vi "box viosion.vi"(8 "Error In":errorcluster) -> (0 "error out":errorcluster, 2 "Array out":string[][](array[string]))   [LabVIEW 2019]
panel:
  out "Array":cluster{i32, i32}[][](array[cluster])
  out "Image":T1(plugin-control)
  out "Image Out":T1(plugin-control)
  # "black\ngreen\nblue\nred"
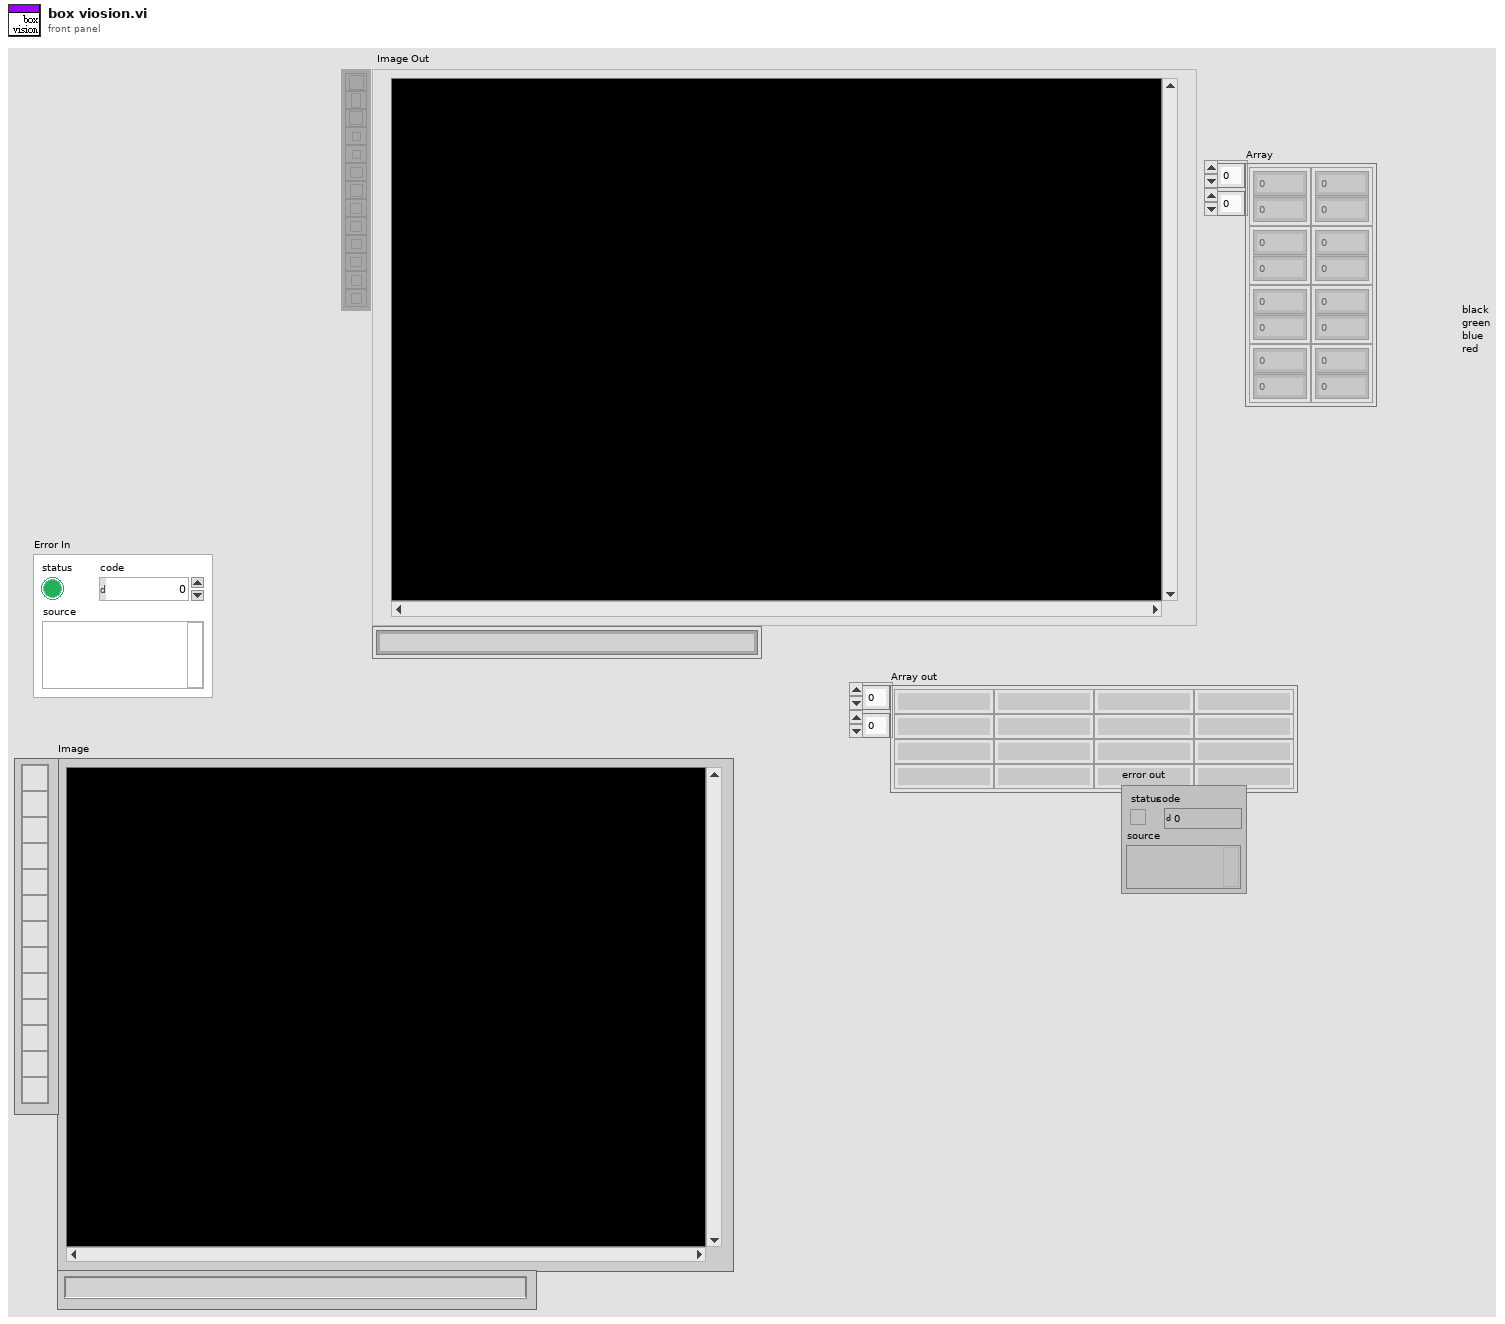
[diagram p1: front panel]
types:
  T1 = typedef "IMAQ Image.ctl" = refnum<image>
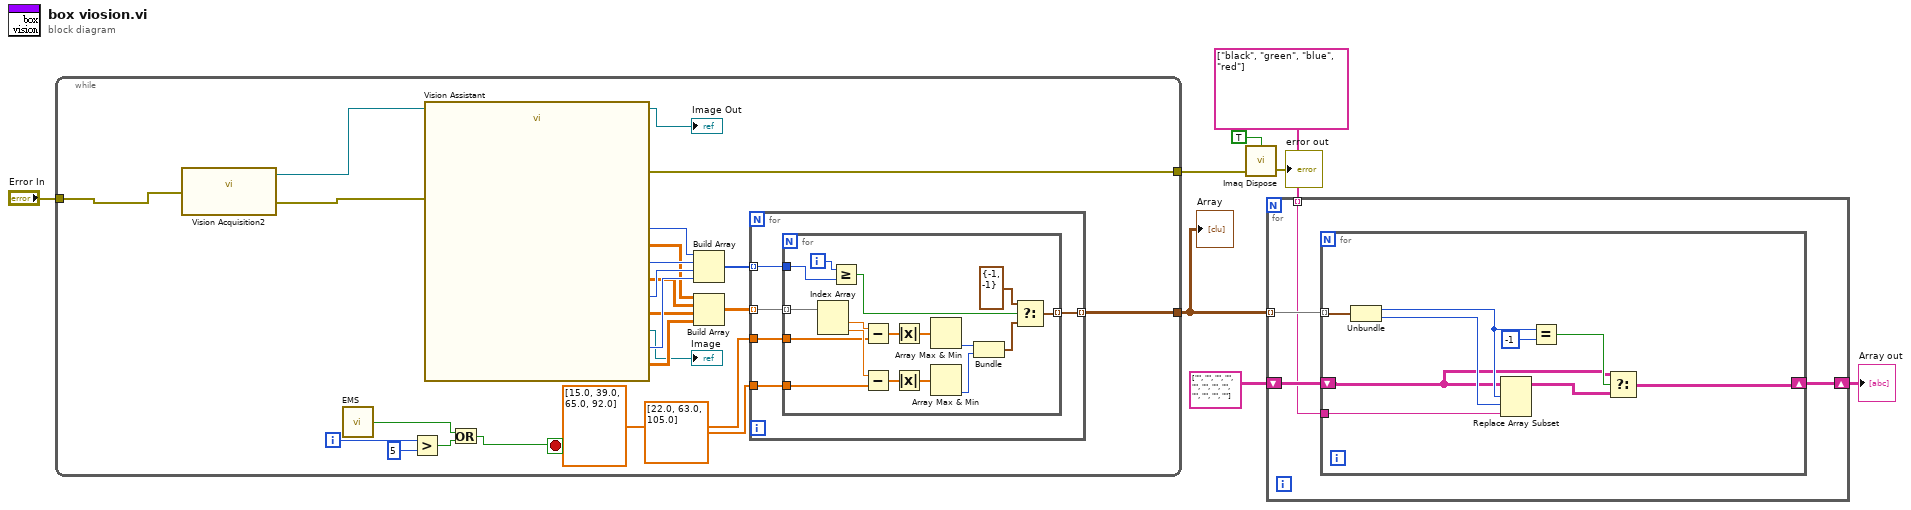
[diagram p0: block diagram]
diagram:
  n1 = while {
    tunnel: [w24] -> w1
    tunnel: "Error In" -> [w15]
    tunnel: [w18] -> w7
    i -> [w13]
    stop <- w9 stop-if-true
    n2 = call "Vision Acquisition2"("error in"=w15) -> ("Image Out"=w16:T1, "error out"=w14:errorcluster)  [unwired: 25 in]
    n3 = call "EMS.vi"() -> ("A/DIO4 (Pin 19)"=w10:bool)
    n4 = Greater?(x=w13, y=5) -> (0:w11:bool)
    n5 = call "Vision Assistant"("Image In"=w16, "error in"=w14) -> ("Image Buffer (Image Buffer 5)"=→"Image":T1, "Particle Measurements (Pixels) (Red)"=w26:dbl[][], "Number of Particles (Red)"=w31:i32, "Image Out"=→"Image Out":T1, "Number of Particles (Black)"=w32:i32, "Particle Measurements (Pixels) (Black)"=w28:dbl[][], "Number of Particles (Green)"=w29:i32, "Particle Measurements (Pixels) (Green)"=w27:dbl[][], "Number of Particles (Blue)"=w30:i32, "Particle Measurements (Pixels) (Blue)"=w25:dbl[][], "error out"=w24:errorcluster)  [unwired: 15 in]
    n6 = Or(x=w10, y=w11) -> (x .or. y?=w9:bool)
    n7 = Build Array(w32, w29, w30, w31) -> (w22:i32[])
    n8 = Build Array(w28, w27, w25, w26) -> (w23:dbl[][][])
    n9 = for {
      tunnel: w23 -> [w37] mode=indexing
      tunnel: w22 -> [w33] mode=indexing
      tunnel: dbl[] [15.0, 39.0, 65.0, 92.0] -> [w36]
      tunnel: dbl[] [22.0, 63.0, 105.0] -> [w35]
      tunnel: [w34] -> w18 mode=indexing
      n10 = for {
        tunnel: w37 -> [w54] mode=indexing
        tunnel: w36 -> [w51]
        tunnel: w35 -> [w50]
        tunnel: [w43] -> w34 mode=indexing
        tunnel: w33 -> [w38]
        i -> [w39]
        n11 = Index Array(array=w54) -> (element #1=w53:dbl, element #2=w52:dbl)  [unwired: 2 in]
        n12 = Greater Or Equal?(x=w39, y=w38) -> (x >= y?=w41:bool)
        n13 = Subtract(x=w53, y=w51) -> (x-y=w49:dbl[])
        n14 = Subtract(x=w52, y=w50) -> (x-y=w48:dbl[])
        n15 = Absolute Value(x=w49) -> (abs(x)=w47:dbl[])
        n16 = Absolute Value(x=w48) -> (abs(x)=w46:dbl[])
        n17 = Array Max & Min(array=w47) -> (min index (indices)=w44:i32)  [unwired: 3 out]
        n18 = Array Max & Min(array=w46) -> (min index (indices)=w45:i32)  [unwired: 3 out]
        n19 = Bundle(w44, w45) -> (w42:cluster{i32, i32})  [unwired: 1 in]
        n20 = Select(t=cluster{i32, i32} {-1, -1} ("output cluster"), s=w41, f=w42) -> (s? t:f=w43:cluster{i32, i32})
      }
    }
  }
  "Array" <- w7
  n21 = call "Imaq Dispose"("All Images? (No)"=TRUE, "error in (no error)"=w1) -> ("error out"=→"error out":errorcluster)  [unwired: 4 in]
  n22 = for {
    tunnel: w7 -> [w58] mode=indexing
    shift-right: [w55] -> w4
    shift-left: string[][] [["", "", ""], ["", "", ""], ["", "", ""], ["", "", ""]] -> [w57]
    tunnel: string[] ["black", "green", "blue", "red"] -> [w56] mode=indexing
    n23 = for {
      tunnel: w58 -> [w67] mode=indexing
      shift-right: [w62] -> w55
      shift-left: w57 -> [w59]
      tunnel: w56 -> [w65]
      n24 = Unbundle(w67) -> (w64:i32, w66:i32)
      n25 = Replace Array Subset(array=w59, new element=w65, index (row)=w64, index (col)=w66) -> (w61:string[][])
      n26 = Equal?(x=w64, y=-1) -> (x = y?=w60:bool)
      n27 = Select(t=w59, s=w60, f=w61) -> (s? t:f=w62:string[][])
    }
  }
  "Array out" <- w4
